vi "Load Structure in VESTA.vi"(10 "Vesta .exe Location":path=path "C:/Program Files (x86)/VESTA/VESTA.exe", 11 "Atomic Structure":T1={"Structure Name"="ATK-generated POSCAR  \r\n", "Lattice vector a"=[6.48, 0.0, 0.0], "Lattice vector b"=[0.0, 6.48, 0.0], "Lattice vector c"=[0.0, 0.0, 32.4], "Atoms Array"=[{"Atom Name"="", "Positions (Direct)"=[[0.0, 0.0, 0.0005805493563561], [0.5, 0.5, 0.0005805493563561], [0.5, 0.0, 0.1012044869316679], [0.0, 0.5, 0.1012044869316679], [0.0, 0.0, 0.201657427297086], [0.5, 0.5, 0.201657427297086], [0.5, 0.0, 0.3022756106216986], [0.0, 0.5, 0.3022756106216986], [0.25, 0.25, 0.3937799251008503], [0.75, 0.75, 0.3937799251008503], [0.75, 0.25, 0.5004577122084005], [0.25, 0.75, 0.5004577122084005], [0.0, 0.0, 0.5916454825280393], [0.5, 0.5, 0.5916454825280393], [0.5, 0.0, 0.6986135219684406], [0.0, 0.5, 0.6986135219684406], [0.0, 0.0, 0.7992442554474246], [0.5, 0.5, 0.7992442554474246], [0.5, 0.0, 0.8999316304227629], [0.0, 0.5, 0.8999316304227629]], "Positions (Cartesian)"=[[0.0, 0.0, 0.0005805493563561], [0.5, 0.5, 0.0005805493563561], [0.5, 0.0, 0.1012044869316679], [0.0, 0.5, 0.1012044869316679], [0.0, 0.0, 0.201657427297086], [0.5, 0.5, 0.201657427297086], [0.5, 0.0, 0.3022756106216986], [0.0, 0.5, 0.3022756106216986], [0.25, 0.25, 0.3937799251008503], [0.75, 0.75, 0.3937799251008503], [0.75, 0.25, 0.5004577122084005], [0.25, 0.75, 0.5004577122084005], [0.0, 0.0, 0.5916454825280393], [0.5, 0.5, 0.5916454825280393], [0.5, 0.0, 0.6986135219684406], [0.0, 0.5, 0.6986135219684406], [0.0, 0.0, 0.7992442554474246], [0.5, 0.5, 0.7992442554474246], [0.5, 0.0, 0.8999316304227629], [0.0, 0.5, 0.8999316304227629]]}, {"Atom Name"="", "Positions (Direct)"=[[0.25, 0.25, 0.0508700657751452], [0.75, 0.75, 0.0508700657751452], [0.75, 0.25, 0.1514314226755048], [0.25, 0.75, 0.1514314226755048], [0.25, 0.25, 0.2516943562152962], [0.75, 0.75, 0.2516943562152962], [0.75, 0.25, 0.356312302565805], [0.25, 0.75, 0.356312302565805], [0.0, 0.0, 0.4497768887256497], [0.5, 0.5, 0.4497768887256497], [0.5, 0.0, 0.553935227460559], [0.0, 0.5, 0.553935227460559], [0.25, 0.25, 0.6478094902292927], [0.75, 0.75, 0.6478094902292927], [0.75, 0.25, 0.7489441399571884], [0.25, 0.75, 0.7489441399571884], [0.25, 0.25, 0.8495690683463202], [0.75, 0.75, 0.8495690683463202], [0.75, 0.25, 0.9502664361665122], [0.25, 0.75, 0.9502664361665122]], "Positions (Cartesian)"=[[0.25, 0.25, 0.0508700657751452], [0.75, 0.75, 0.0508700657751452], [0.75, 0.25, 0.1514314226755048], [0.25, 0.75, 0.1514314226755048], [0.25, 0.25, 0.2516943562152962], [0.75, 0.75, 0.2516943562152962], [0.75, 0.25, 0.356312302565805], [0.25, 0.75, 0.356312302565805], [0.0, 0.0, 0.4497768887256497], [0.5, 0.5, 0.4497768887256497], [0.5, 0.0, 0.553935227460559], [0.0, 0.5, 0.553935227460559], [0.25, 0.25, 0.6478094902292927], [0.75, 0.75, 0.6478094902292927], [0.75, 0.25, 0.7489441399571884], [0.25, 0.75, 0.7489441399571884], [0.25, 0.25, 0.8495690683463202], [0.75, 0.75, 0.8495690683463202], [0.75, 0.25, 0.9502664361665122], [0.25, 0.75, 0.9502664361665122]]}], "# of atoms"=40}) -> ()   [LabVIEW 2010]
uses:
  <vilib>/Utility/sysdir.llb/System Directory Type.ctl
panel:
  out "POSCAR File":string
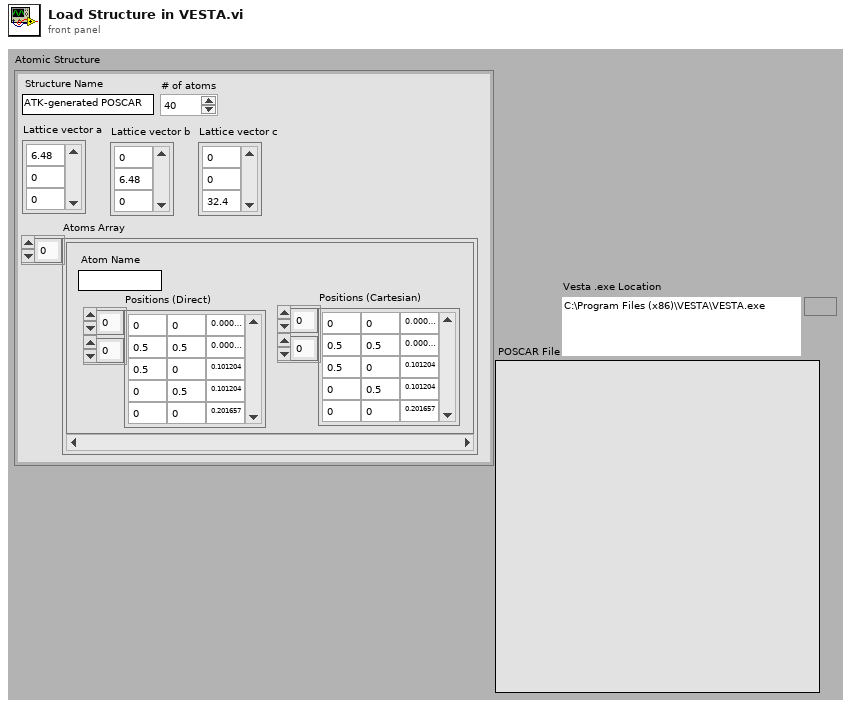
[diagram p1: front panel]
types:
  T1 = cluster{"Structure Name":string, "Lattice vector a":dbl[], "Lattice vector b":dbl[], "Lattice vector c":dbl[], "Atoms Array":cluster{"Atom Name":string, "Positions (Direct)":dbl[][], "Positions (Cartesian)":dbl[][]}[], "# of atoms":i32}
  T2 = typedef "System Directory Type.ctl" = i32
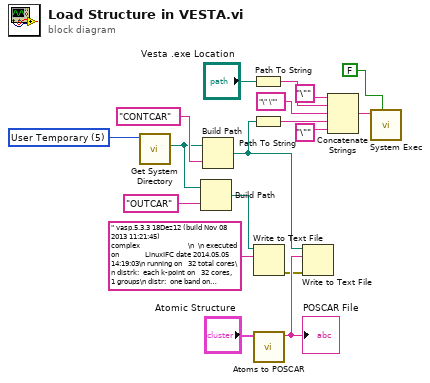
[diagram p0: block diagram]
diagram:
  w1 = T2 5 items=["User Home"=0, "User Desktop"=1, "User Documents"=2, "User Application Data"=3, "User Preferences"=4, "User Temporary"=5, "Public Documents"=6, "Public Application Data"=7, "Public Preferences"=8, "Public Cache"=13, "System Core Libraries"=9, "System Installed Libraries"=10, "Application Files"=11, "Boot Volume Root"=12] ("system directory type")
  n1 = call <vilib>:"Get System Directory.vi"("system directory type"=w1) -> ("system directory"=w15:path)  [unwired: 10 in]
  n2 = Build Path(base path=w15, name or relative path="OUTCAR") -> (appended path=w14:path)
  n3 = Build Path(base path=w15, name or relative path="CONTCAR") -> (appended path=w3:path)
  n4 = Path To String(path="Vesta .exe Location") -> (string=w6:string)
  n5 = Path To String(path=w3) -> (string=w8:string)
  n6 = Write to Text File(file (use dialog)=w14, text=" vasp.5.3.3 18Dez12 (build Nov 08 2013 11:21:45) complex                        \n  \n executed on             LinuxIFC date 2014.05.05  14:19:03\n running on   32 total cores\n distrk:  each k-point on   32 cores,    1 groups\n distr:  one band on NCORES_PER_BAND=   8 cores,    4 groups\n\n\n--------------------------------------------------------------------------------------------------------\n\n\n INCAR:\n POTCAR:   PAW_PBE Cd 06Sep2000                   \n POTCAR:  PAW_PBE Te 08Apr2002                    \n POTCAR:   PAW_PBE Cd 06Sep2000    " ("name or relative path")) -> (error out=w13:errorcluster)  [unwired: 2 in, 2 out]
  n7 = call "Atoms to POSCAR.vi"("Atomic Structure"="Atomic Structure") -> ("POSCAR File"=w18:string)  [unwired: 10 in]
  "POSCAR File" <- w18
  n8 = Write to Text File(file (use dialog)=w3, text=w18, error in=w13) -> ()  [unwired: 1 in, 3 out]
  n9 = Concatenate Strings("\"" ("string"), w6, "\" \"" ("string"), w8, "\"" ("string")) -> (w5:string)
  n10 = call <vilib>:"System Exec.vi"("wait until completion? (T)"=FALSE, "command line"=w5) -> ()  [unwired: 6 in, 4 out]
